vi "Test - Current Consumption.vi"(8 "error in (no error)":errorcluster) -> (0 "error out":errorcluster)   [LabVIEW 2020]
uses:
  Library - Test Executive.llb/Test Executive.lvlib
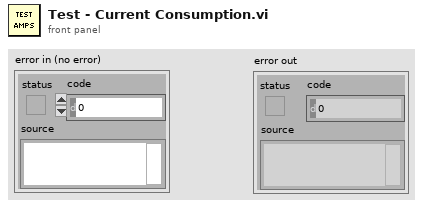
[diagram p1: front panel]
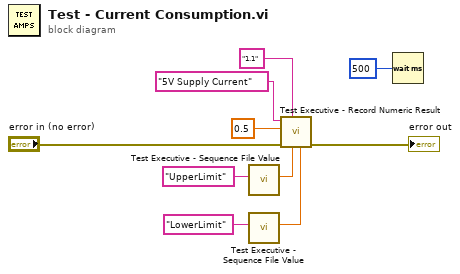
[diagram p0: block diagram]
diagram:
  n1 = call "Test Executive - Sequence File Value.vi"("Key"="UpperLimit") -> ("Numeric Value"=w6:dbl)  [unwired: 7 in, 3 out]
  n2 = call "Test Executive - Sequence File Value.vi"("Key"="LowerLimit") -> ("Numeric Value"=w5:dbl)  [unwired: 7 in, 3 out]
  n3 = call "Test Executive - Record Numeric Result.vi"("Lower Limit"=w5, "Upper Limit"=w6, "Test Ref"="1.1", "error in (no error)"="error in (no error)", "Measurement"=0.5, "Test Name"="5V Supply Current") -> ("error out"=→"error out":errorcluster)  [unwired: 5 in]
  n4 = Wait (ms)(milliseconds to wait=u32 500) -> ()  [unwired: 1 out]
